vi "Actor Core.vi"(8 "error in":errorcluster, 11 "RDS Serial Instrument Actor in":refnum<class "RDS Serial Instrument Actor.lvclass">) -> (0 "error out":errorcluster, 3 "Actor out":refnum<class "Actor.lvclass">)   [LabVIEW 2015, in "RDS Abstracts.lvlib" / "RDS Serial Instrument Actor.lvlib" / "RDS Serial Instrument Actor.lvclass"]
doc: "(<B>Filename</B>: Actor Framework.lvlib:Actor.lvclass:Actor Core.vi)\n\nReceives messages to the actor, reacts to them, and initiates any error handling that may shut the actor down.\n\nDescendant classes may override this VI to append parallel tasks for the actor to complete while it handles messages. Overrides use the Call Parent Method node."
uses:
  RDS Serial Instrument Actor.lvclass
  Libraries/RDS Serial Handler/RDS Serial Instrument.lvclass
  <vilib>/ActorFramework/Actor/Actor.lvclass
  RDS Serial Instrument Actor Messages/RDS Serial Handle Frame Msg/RDS Serial Handle Frame Msg.lvclass
  RDS Parent Actor/RDS Parent Actor/RDS Parent Actor.lvclass
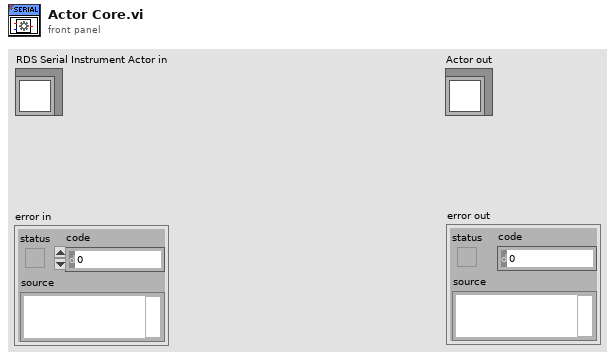
[diagram p1: front panel]
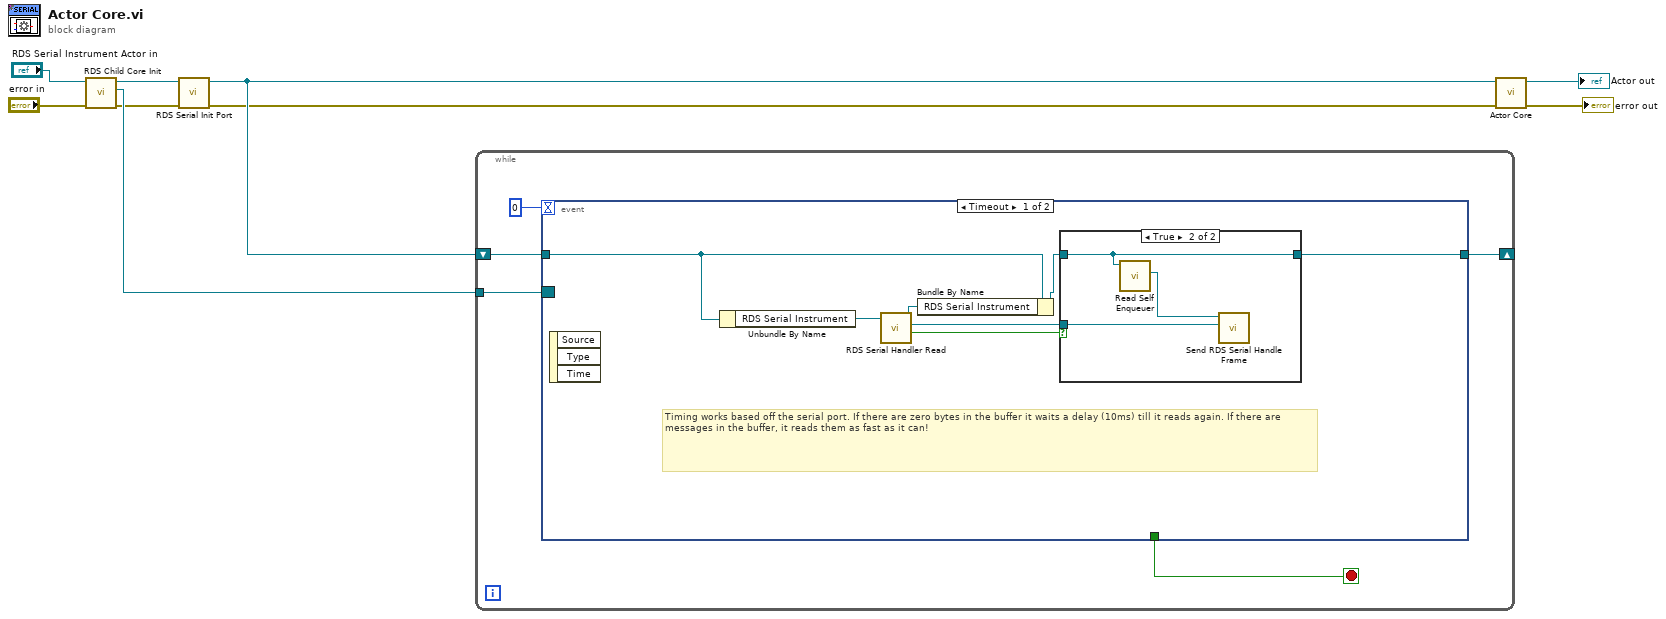
[diagram p0: block diagram]
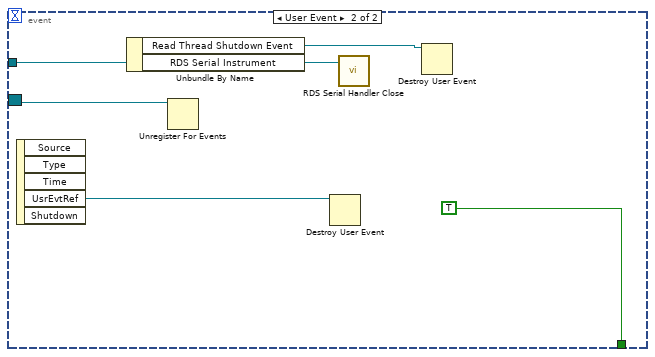
[diagram p3: hidden frame]
diagram:
  n1 = call "RDS Child Core Init.vi"("error in (no error)"="error in", "RDS Parent Actor in"="RDS Serial Instrument Actor in") -> ("error out"=w2:errorcluster, "Event Registration Refnum"=w5:refnum<event-registration>, "RDS Parent Actor out"=w4:refnum<class "RDS Serial Instrument Actor.lvclass">)  [unwired: 6 in, 1 out]
  n2 = call "RDS Serial Init Port.vi"("error in (no error)"=w2, "RDS Serial Instrument Actor in"=w4) -> ("error out"=w1:errorcluster, "RDS Serial Instrument Actor out"=w3:refnum<class "RDS Serial Instrument Actor.lvclass">)  [unwired: 8 in]
  n3 = while {
    shift-right: [w14] -> _
    shift-left: w3 -> [w13]
    tunnel: w5 -> [w10]
    stop <- w11 stop-if-true
    n4 = event shown="[0] Timeout" {
      selector: w10 -> [_ w30]
      dyn-events: _ -> [_ _]
      timeout: 0 -> [_ _]
      tunnel: [w20 _] -> w14
      tunnel: w13 -> [w16 w28]
      tunnel: [_ TRUE] -> w11
      event Timeout {
        # "Timing works based off the serial port. If there are zero bytes in the buffer it waits a delay (10ms) till it reads again. If there are messages in the buffer, it reads them as fast as it can!"
        n5 = event-data() -> ()  [unwired: 1 in, 3 out]
        n6 = Unbundle By Name(w16) -> ("RDS Serial Instrument"=w21:refnum<class "RDS Serial Instrument.lvclass">)
        n7 = call "RDS Serial Handler Read.vi"("RDS Serial Instrument in"=w21) -> ("Data Valid?"=w19:bool, "RDS Serial Frame out"=w18:refnum<class "RDS Serial Frame.lvclass">, "RDS Serial Instrument out"=w17:refnum<class "RDS Serial Instrument.lvclass">)  [unwired: 7 in, 1 out]
        n8 = Bundle By Name(cluster=w16, "RDS Serial Instrument"=w17) -> (w15:refnum<class "RDS Serial Instrument Actor.lvclass">)
        n9 = case shown="True" w19 {
          tunnel: [w22 w25] -> w20
          tunnel: w15 -> [w22 w25]
          tunnel: w18 -> [_ w23]
          frame False {
          }
          frame True {
            n10 = call <vilib>:"Read Self Enqueuer.vi"("Actor"=w25) -> ("Self Enqueuer"=w24:refnum<class "Message Enqueuer.lvclass">)  [unwired: 10 in]
            n11 = call "Send RDS Serial Handle Frame.vi"("RDS Serial Frame"=w23, "Message Enqueuer in"=w24) -> ()  [unwired: 8 in, 2 out]
          }
        }
      }
      event User Event {
        n12 = event-data() -> ("UsrEvtRef"=w29:refnum<user-event>)  [unwired: 1 in, 4 out]
        n13 = Unbundle By Name(w28) -> ("Read Thread Shutdown Event"=w26:refnum<user-event>, "RDS Serial Instrument"=w27:refnum<class "RDS Serial Instrument.lvclass">)
        n14 = Unregister For Events(event registration refnum=w30) -> ()  [unwired: 1 in, 1 out]
        n15 = Destroy User Event(user event=w29) -> ()  [unwired: 1 in, 1 out]
        n16 = call "RDS Serial Handler Close.vi"("RDS Serial Instrument in"=w27) -> ()  [unwired: 9 in, 2 out]
        n17 = Destroy User Event(user event=w26) -> ()  [unwired: 1 in, 1 out]
      }
    }
  }
  n18 = call-parent "Actor Core.vi"("error in"=w1, "Actor in"=w3) -> ("error out"=→"error out":errorcluster, "Actor out"=→"Actor out":refnum<class "Actor.lvclass">)  [unwired: 8 in]
